vi "Prepare LV to Use Icon Editor Source.vi"   [LabVIEW 2020]
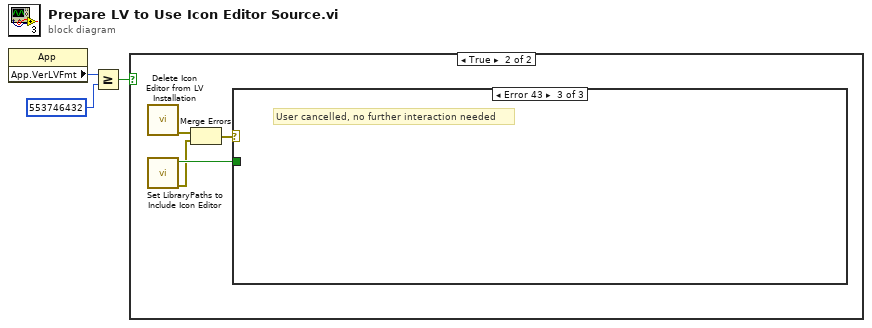
[diagram p0: block diagram]
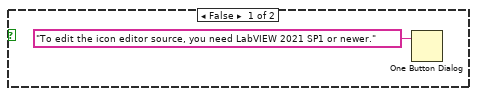
[diagram p2: hidden frame]
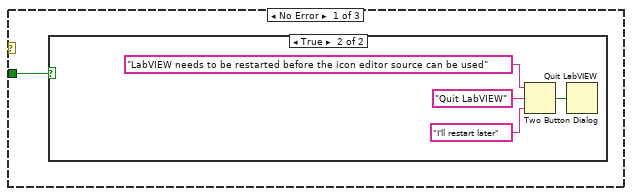
[diagram p3: hidden frame]
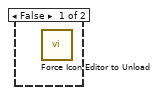
[diagram p4: hidden frame]
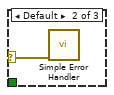
[diagram p5: hidden frame]
diagram:
  n1 = property class="App"() -> ("App.VerLVFmt"=w3:i32)  [unwired: 2 in, 2 out]
  n2 = Greater Or Equal?(x=w3, y=553746432 ("Application:Version As Integer")) -> (x >= y?=w1:bool)
  n3 = case shown="True" w1 {
    frame False {
      n4 = One Button Dialog(message="To edit the icon editor source, you need LabVIEW 2021 SP1 or newer.") -> ()  [unwired: 1 in, 1 out]
    }
    frame True {
      n5 = call "Delete Icon Editor from LV Installation.vi"() -> ("error out"=w7:errorcluster)  [unwired: 10 in, 1 out]
      n6 = call "Set LibraryPaths to Include Icon Editor.vi"() -> ("error out"=w5:errorcluster, "config modified?"=w8:bool)  [unwired: 10 in]
      n7 = Merge Errors(w7, w5) -> (w6:errorcluster)
      n8 = case shown="Error 43" w6 {
        selector: w6 -> [_ w14 _]
        tunnel: w8 -> [w9 _ _]
        frame No Error {
          n9 = case shown="True" w9 {
            frame False {
              n10 = call "Force Icon Editor to Unload.vi"() -> ()  [unwired: 12 in]
            }
            frame True {
              n11 = Two Button Dialog(message="LabVIEW needs to be restarted before the icon editor source can be used", 1:"I'll restart later" ("F button name (\"Cancel\")"), 2:"Quit LabVIEW" ("T button name (\"OK\")")) -> (T button?=w13:bool)
              n12 = Quit LabVIEW(quit? (T)=w13) -> ()
            }
          }
        }
        frame Default {
          n13 = call <vilib>:"Simple Error Handler.vi"("error in (no error)"=w14) -> ()  [unwired: 4 in, 5 out]
        }
        frame Error {
          # "User cancelled, no further interaction needed"
        }
      }
    }
  }
